vi "E_Hole_Input.vi"(4 "error in (no error)":errorcluster, 5 "Measured origin x,y":dbl[](array[numeric])=[0.83, 0.79], 6 "Element In":T5, 7 "Outputmode":u16(ring) items=["Get Path", "Make Layout", "Create TRJs"]) -> (0 "error out":errorcluster, 1 "Init Cluster":T3, 2 "TRJs":T6, 3 "Elements Out":T4(array[cluster]))   [LabVIEW 2009]
panel:
  out "output cluster":T1
  in  "Tab Control":enum32{"machining parameter", "Output"}(tab)=enum."Output"
  in  "XY Line Arc Trajectory":T2={"Velocity (units/s)"=0.5, "Acceleration (unts/s2)"=20.0, "Number of times of execution"=1} {"Acceleration (unts/s2)" format="%.6f"; "Velocity (units/s)" format="%.6f"; "Number of times of execution" format="%.6f"}
  in  "Depth of the hole":dbl=4.0
  in  "change of radus":dbl=0.01
  in  "ablation rate":dbl=0.01
  in  "OR":dbl=0.4
  in  "Center of the hole from bottom edge":dbl=2.35
  in  "Center of the hole  from left edge":dbl=9.9
  in  "IR":dbl
  in  "stop":bool
  in  "Type":i32=3
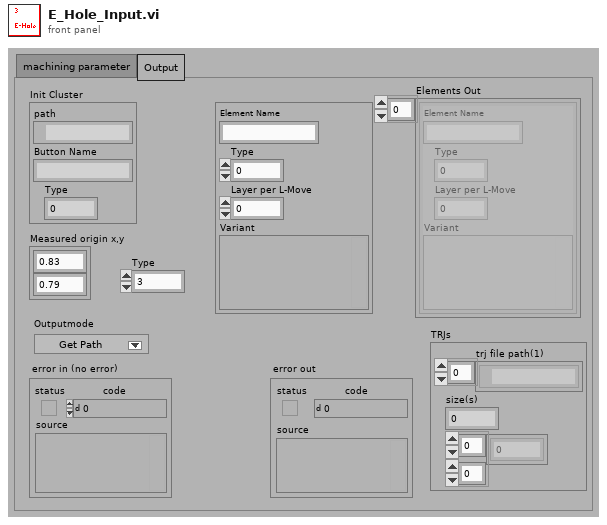
[diagram p1: front panel]
types:
  T1 = cluster{"IR":dbl, "Center of the hole  from left edge":dbl, "Center of the hole from bottom edge":dbl, "OR":dbl, "ablation rate":dbl, "change of radus":dbl, "Depth of the hole":dbl, "XY Line Arc Trajectory":cluster{"Velocity (units/s)":dbl, "Acceleration (unts/s2)":dbl, "Number of times of execution":i32}}
  T2 = cluster{"Velocity (units/s)":dbl, "Acceleration (unts/s2)":dbl, "Number of times of execution":i32}
  T3 = cluster{"path":path, "Button Name":string, "Type":i32}
  T4 = cluster{"Element Name":string, "Type":i32, "Layer per L-Move":i32, "Variant":variant}[]
  T5 = cluster{"Element Name":string, "Type":i32, "Layer per L-Move":i32, "Variant":variant}
  T6 = cluster{"trj file path(1)":path[], "size(s)":i32, dbl[][]}
  T7 = cluster{"Element Name":string, "Value":i32, "Layer per L-Move":i32, "Variant":variant}
  T8 = cluster{"Element Name":string, "Value":i32, "Layer per L-Move":i32, "Variant":variant}[]
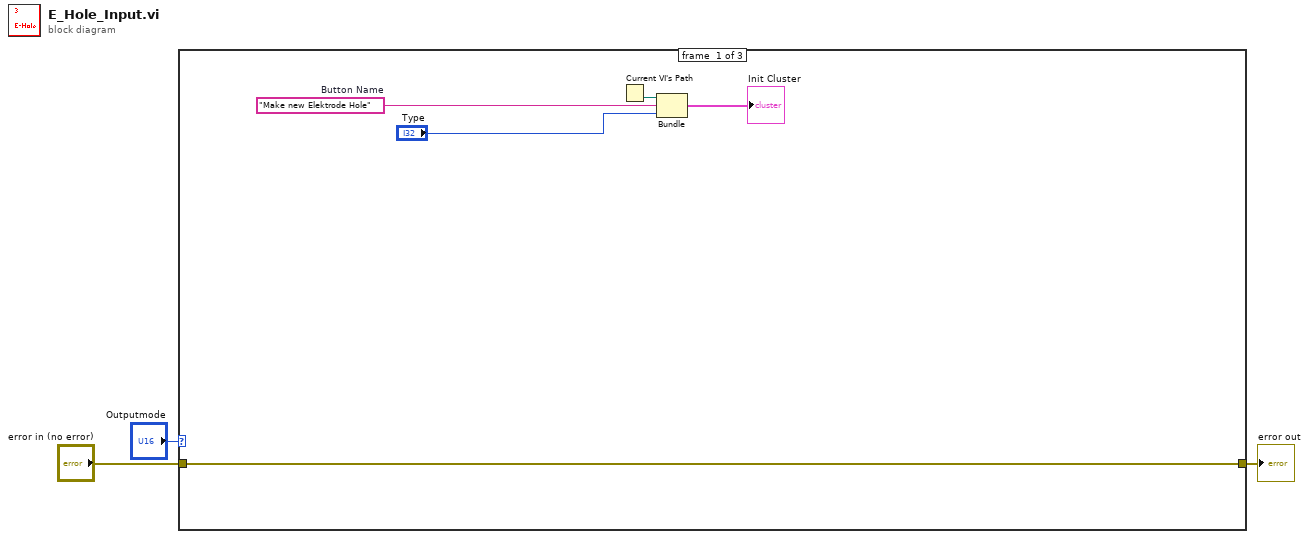
[diagram p0: block diagram]
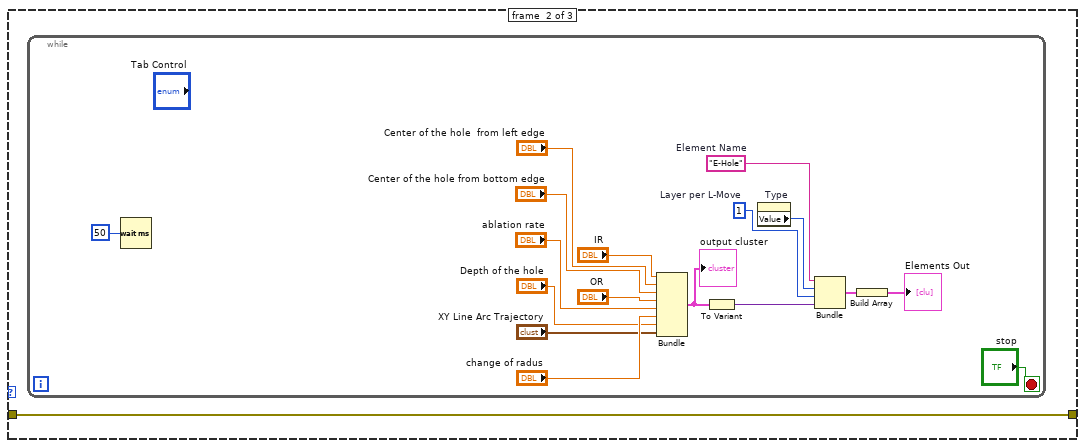
[diagram p2: hidden frame]
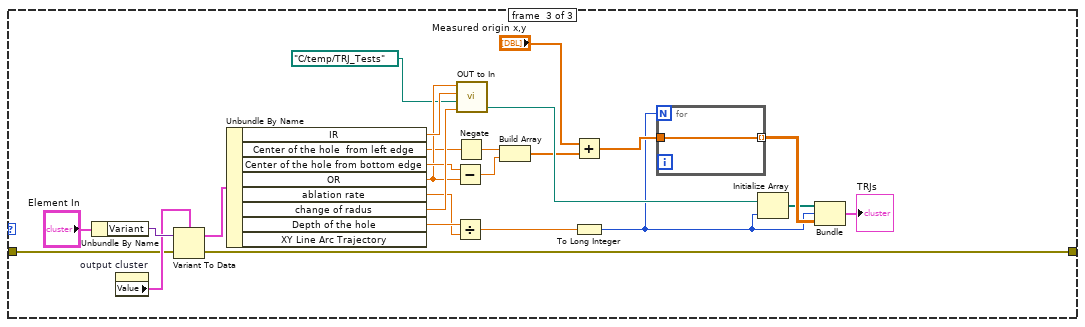
[diagram p3: hidden frame]
diagram:
  n1 = case shown="2" "Outputmode" {
    tunnel: "error in (no error)" -> [w4 w9 w48]
    tunnel: [w4 w9 w28] -> w1
    frame #0 {
      w6 = "Make new Elektrode Hole"  # Button Name
      n2 = Current VI's Path() -> (path=w5:path)
      n3 = Bundle("path"=w5, "Button Name"=w6, "Type"="Type") -> (→"Init Cluster":T3)  [unwired: 1 in]
    }
    frame #1 {
      n4 = while {
        stop <- "stop" stop-if-true
        w15 = 1  # Layer per L-Move
        w12 = "E-Hole"  # Element Name
        n5 = Wait (ms)(milliseconds to wait=u32 50) -> ()  [unwired: 1 out]
        n6 = Bundle("IR"="IR", "Center of the hole  from left edge"="Center of the hole  from left edge", "Center of the hole from bottom edge"="Center of the hole from bottom edge", "OR"="OR", "ablation rate"="ablation rate", "change of radus"="change of radus", "Depth of the hole"="Depth of the hole", "XY Line Arc Trajectory"="XY Line Arc Trajectory") -> (w11:T1)  [unwired: 1 in]
        "output cluster" <- w11
        n7 = To Variant(anything=w11) -> (Variant=w13:variant)
        n8 = property on="Type" class="DigNum (strict)"() -> ("Value"=w10:i32)  [unwired: 2 in, 2 out]
        n9 = Bundle("Element Name"=w12, "Value"=w10, "Layer per L-Move"=w15, "Variant"=w13) -> (w14:T7)  [unwired: 1 in]
        n10 = Build Array(w14) -> (→"Elements Out":T8)
      }
    }
    frame #2 {
      n11 = Unbundle By Name("Element In") -> ("Variant"=w50:variant)
      n12 = property on="output cluster" class="Clust (strict)"() -> ("Value"=w49:T1)  [unwired: 2 in, 2 out]
      n13 = Variant To Data(error in=w48, Variant=w50, type=w49) -> (error out=w28:errorcluster, data=w47:T1)
      n14 = Unbundle By Name(w47) -> ("IR"=w46:dbl, "Center of the hole  from left edge"=w38:dbl, "Center of the hole from bottom edge"=w41:dbl, "OR"=w40:dbl, "ablation rate"=w42:dbl, "change of radus"=w45:dbl, "Depth of the hole"=w43:dbl)  [unwired: 1 out]
      n15 = Subtract(x=w41, y=w40) -> (x-y=w39:dbl)
      n16 = Divide(x=w43, y=w42) -> (x/y=w33:dbl)
      n17 = Negate(x=w38) -> (-x=w37:dbl)
      n18 = call "OUT to In.vi"("OD"=w40, "IO"=w46, "file (use dialog)"=path "C:/temp/TRJ_Tests", "y"=w45) -> ("appended path"=w44:path)  [unwired: 4 out]
      n19 = Build Array(w37, w39) -> (w35:dbl[])
      n20 = Add(x="Measured origin x,y", y=w35) -> (x+y=w34:dbl[])
      n21 = To Long Integer(number=w33) -> (32bit integer=w31:i32)
      n22 = for {
        N: w31 -> [_]
        tunnel: w34 -> [w52]
        tunnel: [w52] -> w32 mode=indexing
      }
      n23 = Initialize Array(w44, w31) -> (w30:path[])
      n24 = Bundle(w30, w31, w32) -> (→"TRJs":cluster{path[], i32, dbl[][]})  [unwired: 1 in]
    }
  }
  "error out" <- w1
